vi "Test 2.vi"(8 "error in (no error)":errorcluster, 11 "Test Case In":refnum<class "Tests.lvclass">) -> (0 "error out":errorcluster, 3 "Test Case Out":refnum<class "Tests.lvclass">)   [LabVIEW 2021, in "Tests.lvclass"]
uses:
  Tests.lvclass
  Tests.lvclass/Tests.ctl
  4993e8ee-a06a-463a-9684-69129f64d5ce.vi
  Proto/Proto.lvclass
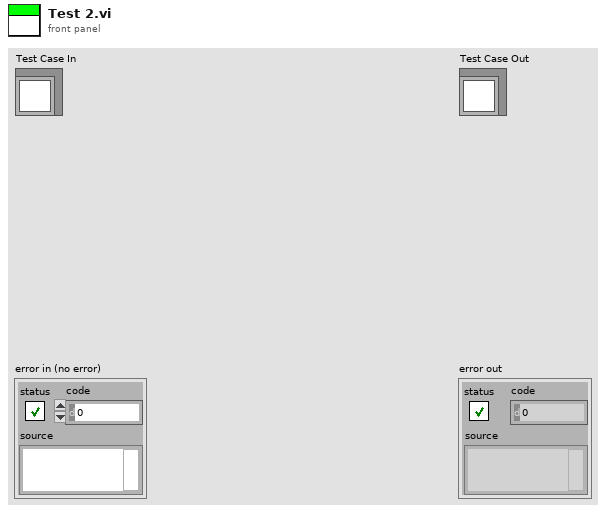
[diagram p1: front panel]
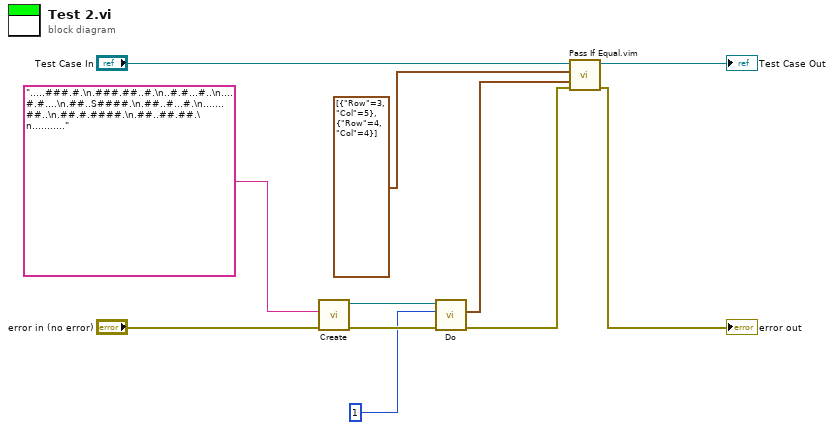
[diagram p0: block diagram]
diagram:
  n1 = call "Create.vi"("error in (no error)"="error in (no error)", "Input"=".....###.#.\n.###.##..#.\n..#.#...#..\n....#.#....\n.##..S####.\n.##..#...#.\n.......##..\n.##.#.####.\n.##..##.##.\n...........") -> ("error out"=w7:errorcluster, "Proto"=w5:refnum<class "Proto.lvclass">)  [unwired: 8 in]
  n2 = call "Do.vi"("error in (no error)"=w7, "Steps"=1, "Proto in"=w5) -> ("error out"=w6:errorcluster, "Possible Coords"=w2:cluster{"Row":i32, "Col":i32}[])  [unwired: 6 in, 1 out]
  n3 = call "Pass If Equal.vim"("error in (no error)"=w6, "Actual"=w2, "Expected"=cluster{"Row":i32, "Col":i32}[] [{"Row"=3, "Col"=5}, {"Row"=4, "Col"=4}] ("Possible Coords"), "LUnit Test Case In"="Test Case In") -> ("error out"=→"error out":errorcluster, "LUnit Test Case Out"=→"Test Case Out":refnum<class "Tests.lvclass">)  [unwired: 6 in]
